vi "GPIO Init.vi"(7 "GPIO #":T3=-1, 8 "error in (no error)":errorcluster, 9 "GPIO Pull (None)":T2, 10 "GPIO Direction":T1, 11 "VisaComms in":refnum<class "VisaComms.lvclass">) -> (0 "error out":errorcluster, 3 "VisaComms out":refnum<class "VisaComms.lvclass">)   [LabVIEW 2024, in "CTI.lvlib" / "VisaComms.lvclass"]
uses:
  VisaComms.lvclass
  GPIO Number.ctl
  GPIO Pull.ctl
  GPIO Direction.ctl
  CTI.lvlib
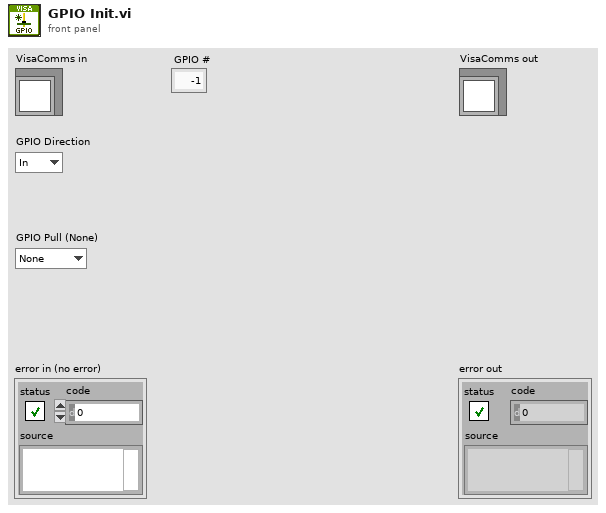
[diagram p1: front panel]
types:
  T1 = typedef "CTI.lvlib/GPIO Direction.ctl" = enum16{"In", "Out"}
  T2 = typedef "CTI.lvlib/GPIO Pull.ctl" = enum16{"None", "Up", "Down", "Both"}
  T3 = typedef "CTI.lvlib/GPIO Number.ctl" = i8
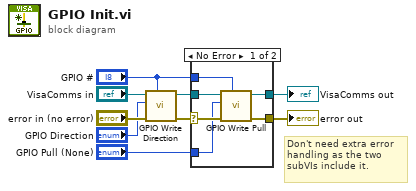
[diagram p0: block diagram]
diagram:
  # "Don't need extra error handling as the two subVIs include it."
  n1 = call-dynamic "GPIO Write Direction.vi"("GPIO #"="GPIO #", "error in (no error)"="error in (no error)", "GPIO Direction"="GPIO Direction", "FirmwareComms in"="VisaComms in") -> ("error out"=w6:errorcluster, "FirmwareComms out"=w7:refnum<class "VisaComms.lvclass">)  [unwired: 6 in]
  n2 = case shown="No Error" w6 {
    selector: w6 -> [w14 w16]
    tunnel: w7 -> [w15 w17]
    tunnel: "GPIO Pull (None)" -> [w13 _]
    tunnel: "GPIO #" -> [w12 _]
    tunnel: [w11 w17] -> w4
    tunnel: [w10 w16] -> w3
    frame No Error {
      n3 = call-dynamic "GPIO Write Pull.vi"("GPIO #"=w12, "error in (no error)"=w14, "GPIO Pull"=w13, "FirmwareComms in"=w15) -> ("error out"=w10:errorcluster, "FirmwareComms out"=w11:refnum<class "VisaComms.lvclass">)  [unwired: 6 in]
    }
    frame Error {
    }
  }
  "error out" <- w3
  "VisaComms out" <- w4
